vi "Uninstall Project.vi"() -> ()   [LabVIEW 2011, in "LVH-Toolbox.lvlib" / "LVH-Build-Tools.lvlib"]
uses:
  LVH-Build-Tools.lvlib
panel:
  out "Deleted Folders":path[](array[path])
  # "Uninstall Source"
  # "1. Run this VI\n2. When prompted select the config.ini file for the project you are working on.  The config.ini should be in the soure root directory.\n3. This VI will remove all source files from the National Instruments\\LabVIEW Directory."
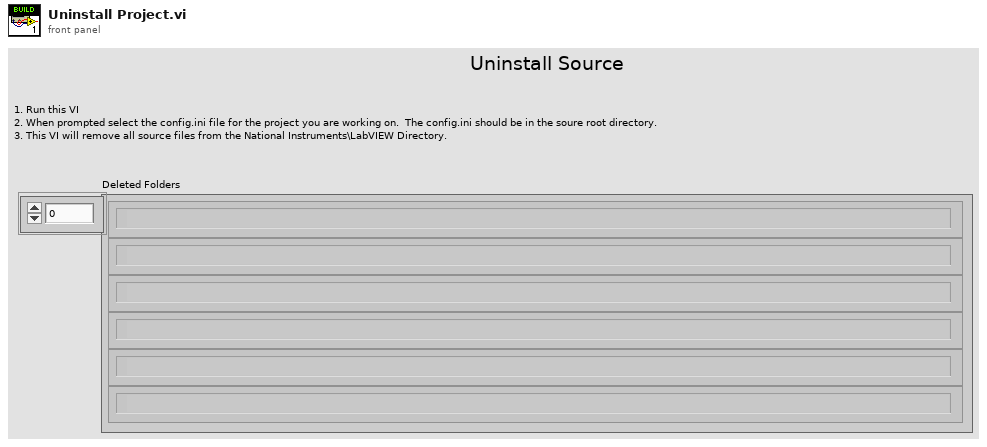
[diagram p1: front panel]
types:
  T1 = typedef "LVH-Toolbox.lvlib/LVH-Build-Tools.lvlib/Configuration.ctl" = cluster{"Source Root":path, "Install Root":string, "Components":string[], "Ignore":string[], "Config Files":path[], "LV Directories":path[], "Install Paths":T2}
  T2 = typedef "LVH-Toolbox.lvlib/LVH-Build-Tools.lvlib/Install Configuration.ctl" = cluster{"LabVIEW Directory":path, "Project Source Config":path}
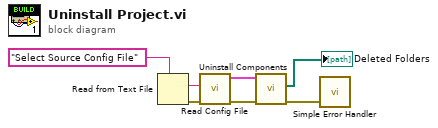
[diagram p0: block diagram]
diagram:
  n1 = Read from Text File(prompt (Open existing file)="Select Source Config File") -> (text=w5:string, error out=w7:errorcluster)  [unwired: 3 in, 2 out]
  n2 = call "Read Config File.vi"("error in (no error)"=w7, "Config File In"=w5) -> ("error out"=w4:errorcluster, "Configuration out"=w3:T1)  [unwired: 8 in]
  n3 = call "Uninstall Components.vi"("error in (no error)"=w4, "Configuration in"=w3) -> ("error out"=w2:errorcluster, "Deleted Components"=→"Deleted Folders":path[])  [unwired: 7 in, 1 out]
  n4 = call <vilib>:"Simple Error Handler.vi"("error in (no error)"=w2) -> ()  [unwired: 4 in, 5 out]
